vi "Handle Error.vi"(8 "error in (no error)":errorcluster, 11 "Broadcast Actor in":refnum<class "Broadcast Actor.lvclass">) -> (0 "error out":errorcluster, 2 "stop actor?":bool=TRUE, 3 "Broadcast Actor out":refnum<class "Broadcast Actor.lvclass">)   [LabVIEW 2015, in "Broadcast Actor.lvlib" / "Broadcast Actor.lvclass"]
doc: "(<B>Filename</B>: Actor Framework.lvlib:Actor.lvclass:Handle Error.vi)\n\nDefines how the actor handles an error that occurred while processing a message. By default, this method does nothing except stop the actor."
uses:
  Broadcast Actor.lvclass
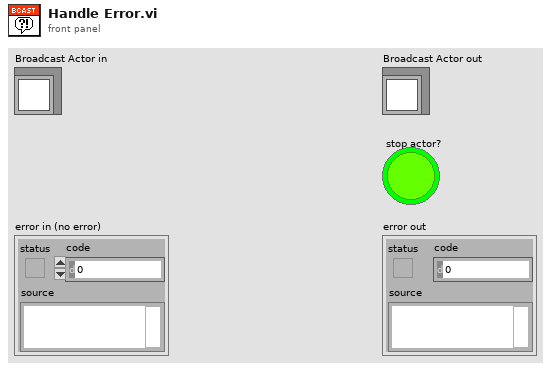
[diagram p1: front panel]
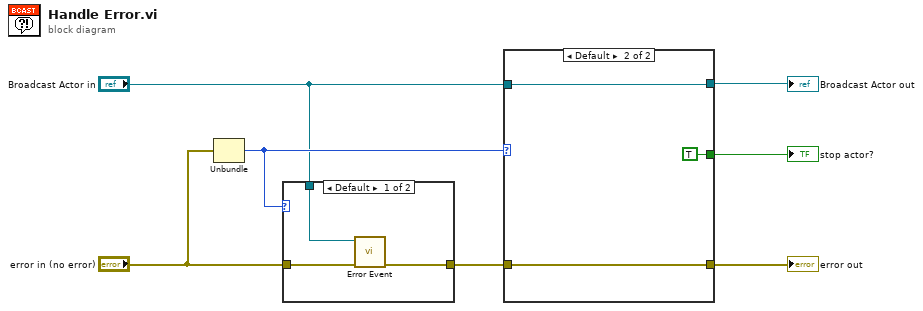
[diagram p0: block diagram]
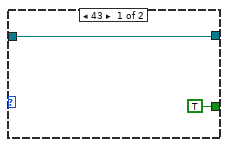
[diagram p3: hidden frame]
diagram:
  n1 = Unbundle("error in (no error)") -> ("code"=w4:i32)  [unwired: 2 out]
  n2 = case shown="Default" w4 {
    tunnel: [w9 w11] -> w2
    tunnel: "error in (no error)" -> [w10 w11]
    tunnel: "Broadcast Actor in" -> [w8 _]
    frame Default {
      n3 = call "Error Event.vi"("error in (no error)"=w10, "Broadcast Actor In"=w8) -> ("error out"=w9:errorcluster)  [unwired: 9 in]
    }
    frame 43 {
    }
  }
  n4 = case shown="Default" w4 {
    tunnel: "Broadcast Actor in" -> [w13 w16]
    tunnel: w2 -> [_ w15]
    tunnel: [_ w15] -> w7
    tunnel: [w13 w16] -> w6
    tunnel: [TRUE TRUE] -> w5
    frame 43 {
    }
    frame Default {
    }
  }
  "Broadcast Actor out" <- w6
  "error out" <- w7
  "stop actor?" <- w5
